vi "NI VeriStand - Remove Calibration.vi"(8 "error in":errorcluster, 10 "Channel Name":string, 11 "Calibration In":T1) -> (0 "error out":errorcluster, 3 "Calibration Out":T1)   [LabVIEW 2020, in "NI_VS Calibration ExecutionAPI.lvlib"]
doc: "Removes the calibration applied to the specified channel."
uses:
  <vilib>/NI VeriStand/Execution/Calibration/NI_VS Calibration ExecutionAPI.lvlib
  <vilib>/NI VeriStand/Execution/Calibration/CalibrationAPI.ctl
  NationalInstruments.VeriStand.ClientAPI
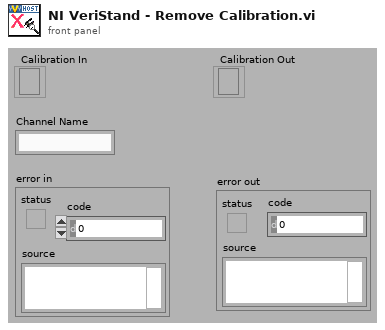
[diagram p1: front panel]
types:
  T1 = typedef "NI_VS Calibration ExecutionAPI.lvlib/CalibrationAPI.ctl" = refnum<k24>
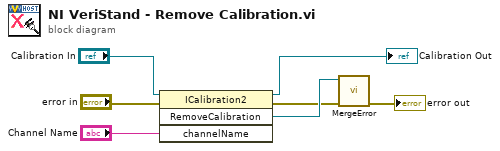
[diagram p0: block diagram]
diagram:
  n1 = invoke class="ICalibration2" method="RemoveCalibration"(reference="Calibration In", error in="error in", "channelName"="Channel Name") -> (reference out=→"Calibration Out":T1, error out=w4:errorcluster, "RemoveCalibration"=w6:refnum<k24>)  [unwired: 1 in, 1 out]
  n2 = call <vilib>:"MergeError.vi"("error in (no error)"=w4, "Error"=w6) -> ("error out"=→"error out":errorcluster)  [unwired: 9 out]
